vi "Recipe_Creator.vi"(8 "Error in":errorcluster) -> (0 "error out 2":errorcluster)   [LabVIEW 2017]
uses:
  <vilib>/Utility/error.llb/DialogType.ctl
  <vilib>/Utility/config.llb/Write Key (U32).vi
  <vilib>/Utility/config.llb/Read Key (U32).vi
  <vilib>/Utility/config.llb/NI_LVConfig.lvlib
  <vilib>/Utility/config.llb/Read Key (Boolean).vi
panel:
  in  "Tabel Update":bool
  in  "Delete Varient":bool
  in  "Varient No":u32
  in  "Varient Name":string(combo)
  out "Table":string[][](table)
  in  "Save Varient":bool
  in  "Close":bool
  out "error out":errorcluster
  out "Machine Name":string
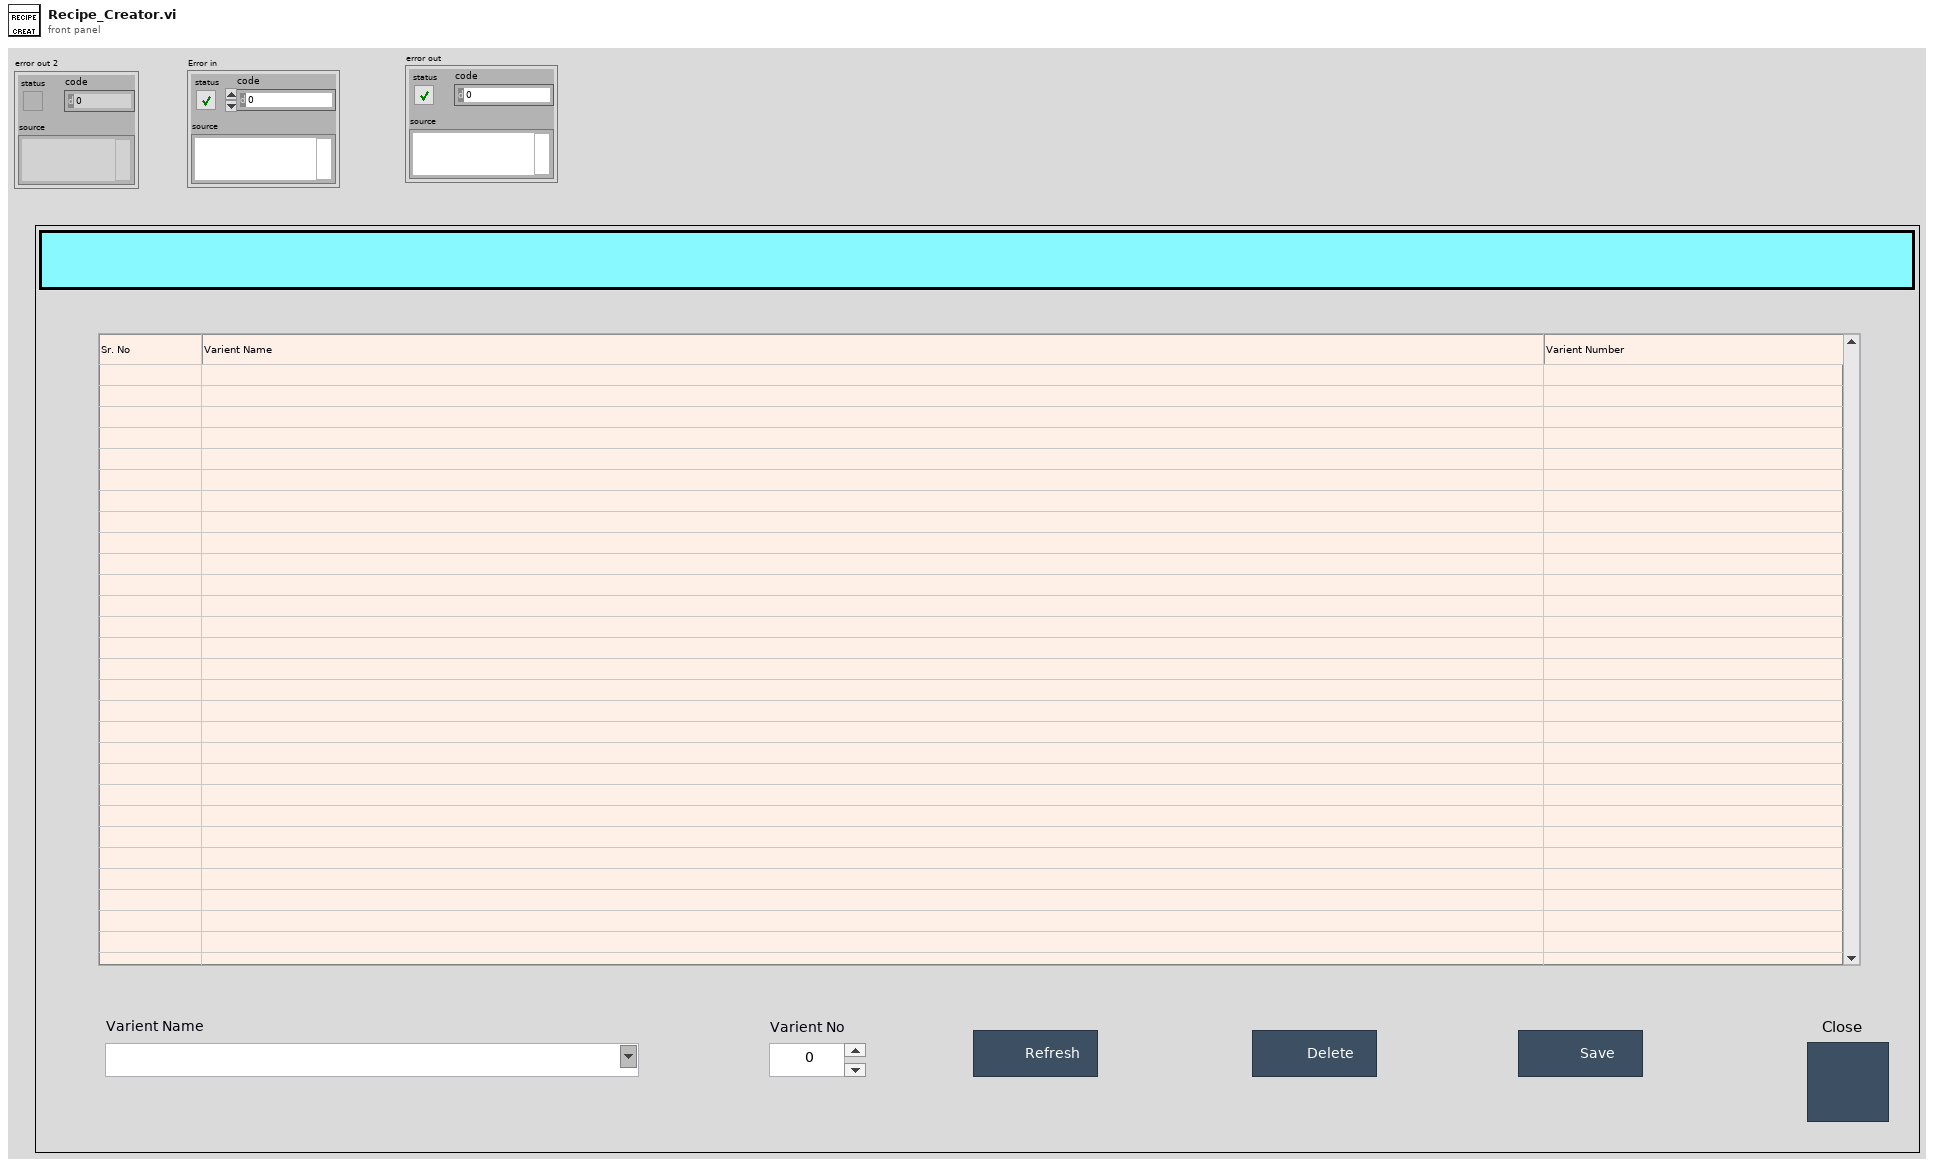
[diagram p1: front panel]
types:
  T1 = enum32{"invalid app kind", "Development System", "Run Time System", "Student Edition", "Embedded LabVIEW", "Evaluation", "Custom"}
  T2 = typedef "NI_LVConfig.lvlib/Config Data RefNum.ctl" = refnum<k1>
  T3 = typedef "DialogType.ctl" = u16
  T4 = enum32{"Invalid", "Standard", "Closed", "Hidden", "Minimized", "Maximized"}
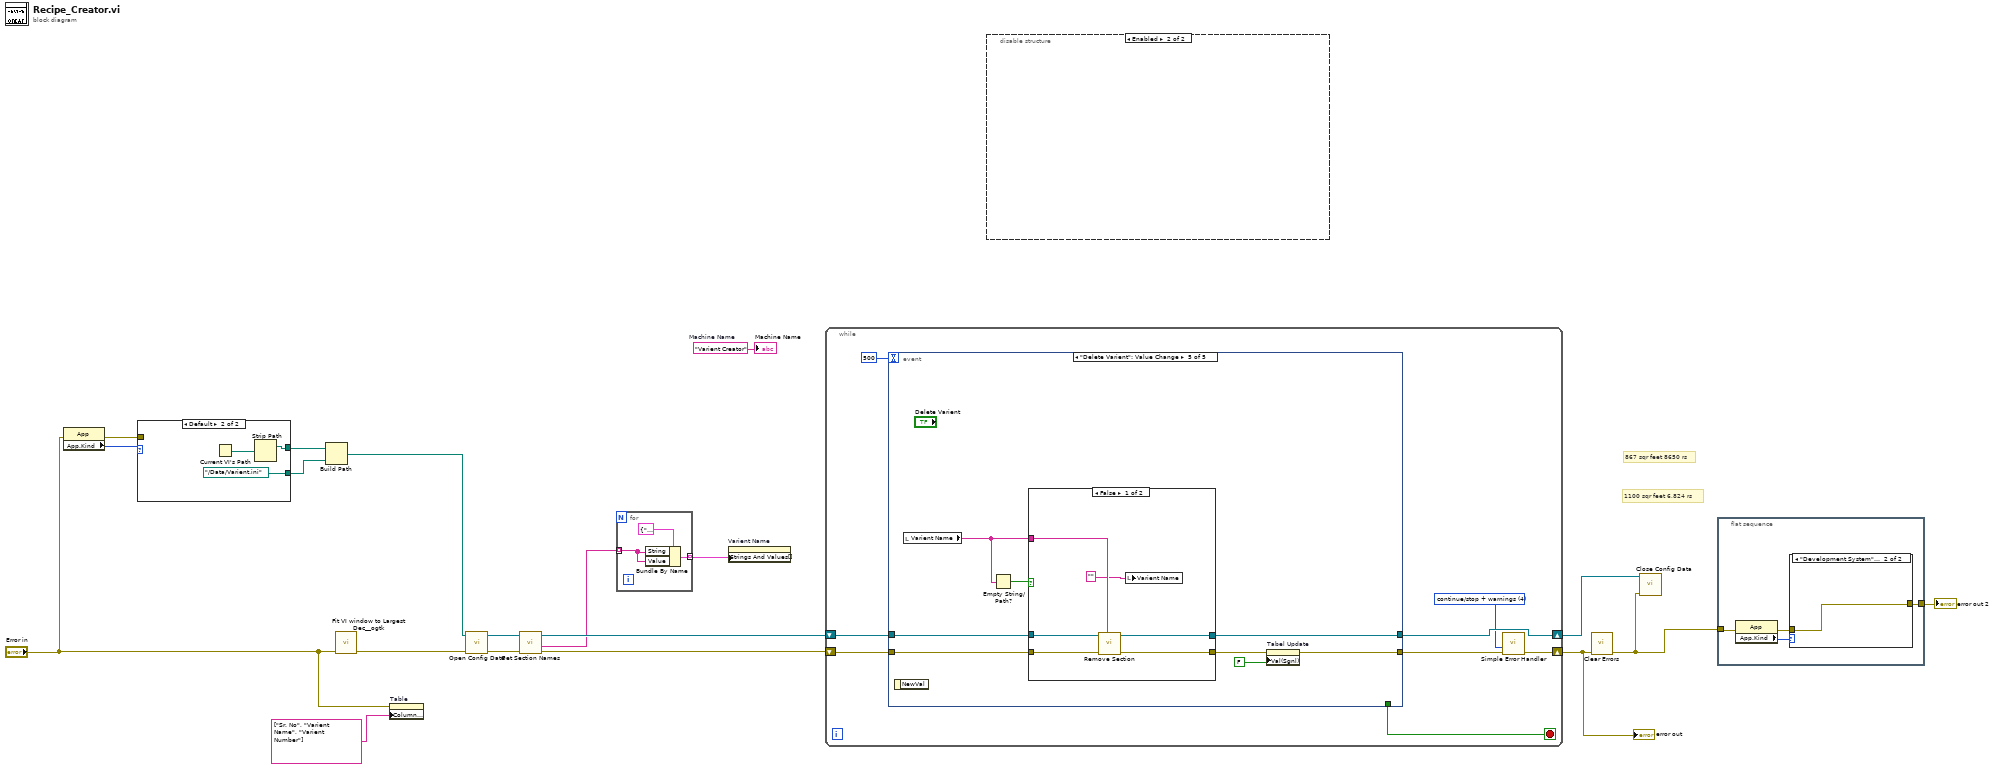
[diagram p0: block diagram]
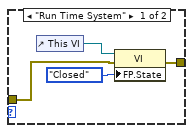
[diagram p2: hidden frame]
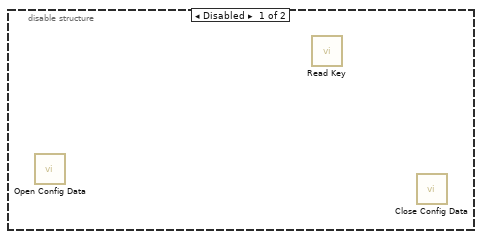
[diagram p3: hidden frame]
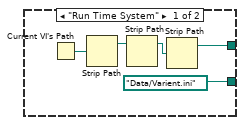
[diagram p4: hidden frame]
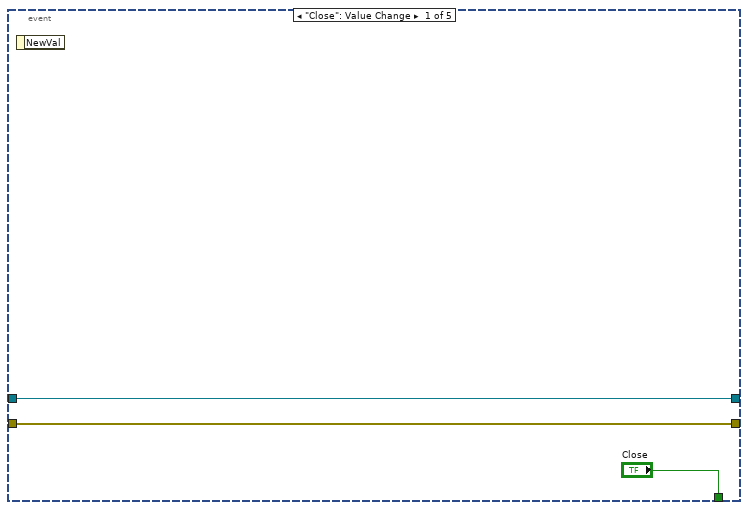
[diagram p5: hidden frame]
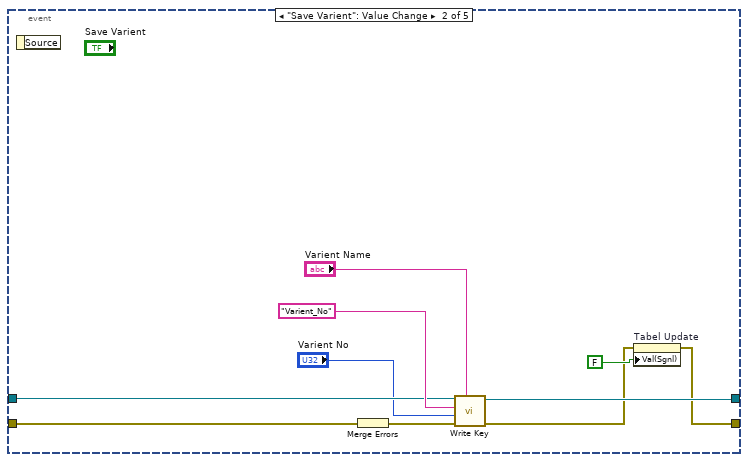
[diagram p6: hidden frame]
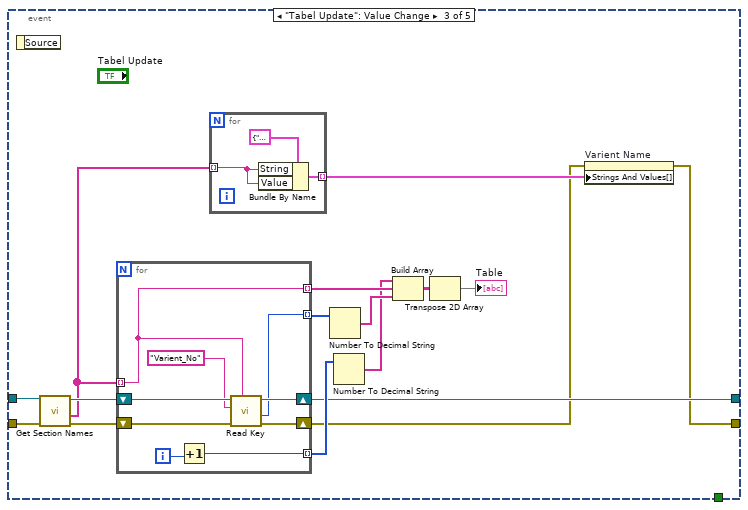
[diagram p7: hidden frame]
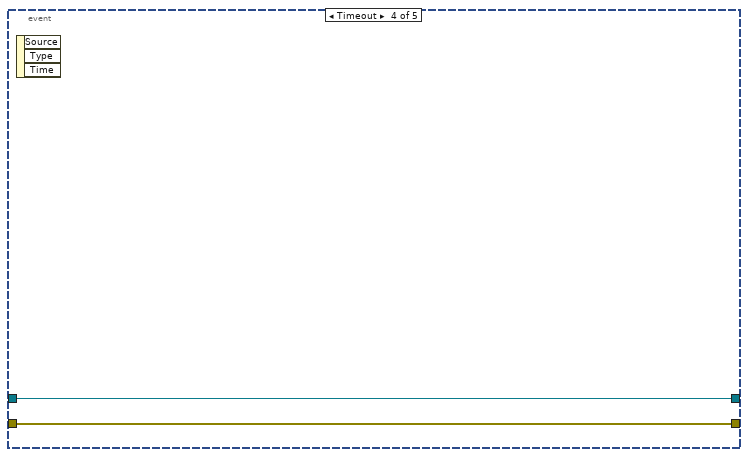
[diagram p8: hidden frame]
diagram:
  w19 = "Varient Creator"  # Machine Name
  # "1100 sqr feet 6,824 rs"
  # "867 sqr feet 8650 rs"
  n1 = property class="App"(error in="Error in") -> (error out=w16:errorcluster, "App.Kind"=w18:T1)  [unwired: 1 in, 1 out]
  n2 = case shown="Default" w18 {
    tunnel: [path "Data/Varient.ini" ("path") path "../Data/Varient.ini" ("path")] -> w17
    tunnel: [w20 w25] -> w15
    tunnel: w16 -> [_ _]
    frame "Run Time System" {
      n3 = Current VI's Path() -> (path=w23:path)
      n4 = Strip Path(path=w23) -> (stripped path=w22:path)  [unwired: 1 out]
      n5 = Strip Path(path=w22) -> (stripped path=w21:path)  [unwired: 1 out]
      n6 = Strip Path(path=w21) -> (stripped path=w20:path)  [unwired: 1 out]
    }
    frame Default {
      n7 = Current VI's Path() -> (path=w26:path)
      n8 = Strip Path(path=w26) -> (stripped path=w25:path)  [unwired: 1 out]
    }
  }
  n9 = Build Path(base path=w15, name or relative path=w17) -> (appended path=w14:path)
  n10 = call <userlib>:"Fit VI window to Largest Dec__ogtk.vi"("error in (no error)"="Error in") -> ("error out"=w11:errorcluster)  [unwired: 5 in, 1 out]
  n11 = property on="Table" class="Tbl (strict)"(error in="Error in", "Column Headers[]"=string[] ["Sr. No", "Varient Name", "Varient Number"]) -> ()  [unwired: 1 in, 2 out]
  n12 = call <vilib>:"Open Config Data.vi"("error in (no error)"=w11, "configuration file path"=w14) -> ("error out"=w9:errorcluster, "refnum"=w10:T2)  [unwired: 7 in, 1 out]
  n13 = call <vilib>:"Get Section Names.vi"("error in (no error)"=w9, "refnum"=w10) -> ("error out"=w8:errorcluster, "section names"=w2:string[], "refnum out"=w3:T2)  [unwired: 7 in]
  n14 = for {
    tunnel: w2 -> [w29] mode=indexing
    tunnel: [w28] -> w1 mode=indexing
    n15 = Bundle By Name(cluster=cluster{"String":string, "Value":string} {"String"="", "Value"=""}, "String"=w29, "Value"=w29) -> (w28:cluster{"String":string, "Value":string})
  }
  n16 = property on="Varient Name" class="CmbBox"("Strings And Values[]"=w1) -> ()  [unwired: 2 in, 2 out]
  n17 = while {
    shift-right: [w34] -> w12
    shift-left: w8 -> [w36]
    shift-right: [w33] -> w4
    shift-left: w3 -> [w32]
    stop <- w38 stop-if-true
    w31 = T3 4 items=["no dialog", "OK message", "continue or stop message", "OK message + warnings", "continue/stop + warnings"] ("type of dialog (OK msg:1)")
    n18 = event shown="[4] \"Delete Varient\": Value Change" {
      selector: _ -> [_ _ _ _ _]
      dyn-events: _ -> [_ _ _ _ _]
      timeout: 500 -> [_ _ _ _ _]
      tunnel: ["Close" _ _ _ _] -> w38
      tunnel: [w40 w42 w52 w81 w82] -> w37
      tunnel: w36 -> [w40 w51 w67 w81 w89]
      tunnel: [w39 w47 w55 w80 w85] -> w33
      tunnel: w32 -> [w39 w48 w59 w80 w86]
      event "Close": Value Change {
        n19 = event-data() -> ()  [unwired: 1 in, 1 out]
      }
      event "Save Varient": Value Change {
        n20 = event-data() -> ()  [unwired: 1 in, 1 out]
        n21 = Merge Errors(w51) -> (w50:errorcluster)
        n22 = call-poly <vilib>:"Write Key.vi"("section"="Varient Name", "error in (no error)"=w50, "value"="Varient No", "key"="Varient_No", "refnum"=w48) -> ("error out"=w43:errorcluster, "refnum out"=w47:T2)  [unwired: 4 in, 1 out]
        n23 = property on="Tabel Update" class="Bool (strict)"(error in=w43, "Val(Sgnl)"=FALSE) -> (error out=w42:errorcluster)  [unwired: 1 in, 1 out]
      }
      event "Tabel Update": Value Change {
        n24 = event-data() -> ()  [unwired: 1 in, 1 out]
        n25 = call <vilib>:"Get Section Names.vi"("error in (no error)"=w67, "refnum"=w59) -> ("error out"=w66:errorcluster, "section names"=w54:string[], "refnum out"=w65:T2)  [unwired: 7 in]
        n26 = for {
          shift-right: [w76] -> w53
          shift-left: w66 -> [w77]
          tunnel: w54 -> [w73] mode=indexing
          tunnel: [w74] -> w64 mode=indexing
          tunnel: [w73] -> w62 mode=indexing
          shift-right: [w78] -> w55
          shift-left: w65 -> [w79]
          tunnel: [w71] -> w58 mode=indexing
          i -> [w72]
          n27 = Increment(x=w72) -> (x+1=w71:i32)
          n28 = call-poly <vilib>:"Read Key.vi"("section"=w73, "error in (no error)"=w77, "key"="Varient_No", "refnum"=w79) -> ("error out"=w76:errorcluster, "value"=w74:u32, "refnum out"=w78:T2)  [unwired: 4 in, 1 out]
        }
        n29 = for {
          tunnel: w54 -> [w69] mode=indexing
          tunnel: [w68] -> w56 mode=indexing
          n30 = Bundle By Name(cluster=cluster{"String":string, "Value":string} {"String"="", "Value"=""}, "String"=w69, "Value"=w69) -> (w68:cluster{"String":string, "Value":string})
        }
        n31 = Number To Decimal String(number=w64) -> (decimal integer string=w63:string[])  [unwired: 1 in]
        n32 = Number To Decimal String(number=w58) -> (decimal integer string=w57:string[])  [unwired: 1 in]
        n33 = Build Array(w57, w62, w63) -> (w61:string[][])
        n34 = Transpose 2D Array(2D array=w61) -> (transposed array=→"Table":string[][])
        n35 = property on="Varient Name" class="CmbBox"(error in=w53, "Strings And Values[]"=w56) -> (error out=w52:errorcluster)  [unwired: 1 in, 1 out]
      }
      event Timeout {
        n36 = event-data() -> ()  [unwired: 1 in, 3 out]
      }
      event "Delete Varient": Value Change {
        n37 = event-data() -> ()  [unwired: 1 in, 1 out]
        n38 = local read "Varient Name"() -> (w87:string)
        n39 = Empty String/Path?(string/path=w87) -> (empty?=w88:bool)
        n40 = case shown="False" w88 {
          tunnel: w87 -> [w95 _]
          tunnel: w89 -> [w94 w97]
          tunnel: [w93 w97] -> w83
          tunnel: [w92 w96] -> w85
          tunnel: w86 -> [w91 w96]
          frame False {
            n41 = call <vilib>:"Remove Section.vi"("section"=w95, "error in (no error)"=w94, "refnum"=w91) -> ("error out"=w93:errorcluster, "refnum out"=w92:T2)  [unwired: 6 in, 1 out]
            n42 = local write "Varient Name"("") -> ()
          }
          frame True {
          }
        }
        n43 = property on="Tabel Update" class="Bool (strict)"(error in=w83, "Val(Sgnl)"=FALSE) -> (error out=w82:errorcluster)  [unwired: 1 in, 1 out]
      }
    }
    n44 = call <vilib>:"Simple Error Handler.vi"("type of dialog (OK msg:1)"=w31, "error in (no error)"=w37) -> ("error out"=w34:errorcluster)  [unwired: 3 in, 4 out]
  }
  "error out" <- w12
  n45 = disable-structure shown="Enabled" {
    frame Disabled {
      n46 = call <vilib>:"Open Config Data.vi"() -> ()  [unwired: 9 in, 3 out]
      n47 = call-poly <vilib>:"Read Key.vi"() -> ()  [unwired: 8 in, 4 out]
      n48 = call <vilib>:"Close Config Data.vi"() -> ()  [unwired: 10 in, 2 out]
    }
    frame Enabled {
    }
  }
  n49 = call <vilib>:"Clear Errors.vi"("error in (no error)"=w12) -> ("error out"=w5:errorcluster)  [unwired: 5 in, 1 out]
  n50 = call <vilib>:"Close Config Data.vi"("error in (no error)"=w5, "refnum"=w4) -> ()  [unwired: 8 in, 2 out]
  n51 = flat-sequence {
    tunnel: [w99] -> w13
    tunnel: w5 -> [w98]
    frame #0 {
      n52 = property class="App"(error in=w98) -> (error out=w100:errorcluster, "App.Kind"=w101:T1)  [unwired: 1 in, 1 out]
      n53 = case shown="\"Development System\", Default" w101 {
        tunnel: w100 -> [w103 w106]
        tunnel: [w102 w106] -> w99
        frame "Run Time System" {
          n54 = control-ref of="This VI"() -> (w105:refnum<vi>)
          n55 = property class="VI"(reference=w105, error in=w103, "FP.State"=T4."Closed" ("Front Panel Window:State")) -> (error out=w102:errorcluster)  [unwired: 1 out]
        }
        frame "Development System", Default {
        }
      }
    }
  }
  "Machine Name" <- w19
  "error out 2" <- w13
